vi "Config DMM.vi"(8 "error in (no error)":errorcluster, 10 "Load DMM Measurement":T1, 11 "IVI Refnum in":refnum<k15>) -> (0 "error out":errorcluster, 3 "IVI Refnum out":refnum<k15>)   [LabVIEW 2021, in "DMM T15.lvlib"]
uses:
  DMM T15.lvlib
  <instrlib>/niDMM/nidmm.llb/niDMM Function.ctl
  <instrlib>/niDMM/nidmm.llb/niDMM Configure Measurement Digits.vi
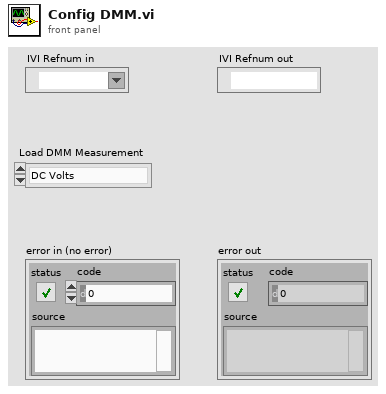
[diagram p1: front panel]
types:
  T1 = typedef "niDMM Function.ctl" = enum16{"DC Volts", "AC Volts", "DC Current", "AC Current", "2-wire Resistance", "4-wire Resistance", "Diode", "Frequency", "Period", "AC Volts DC Coupled", "Capacitance", "Inductance", "Temperature"}
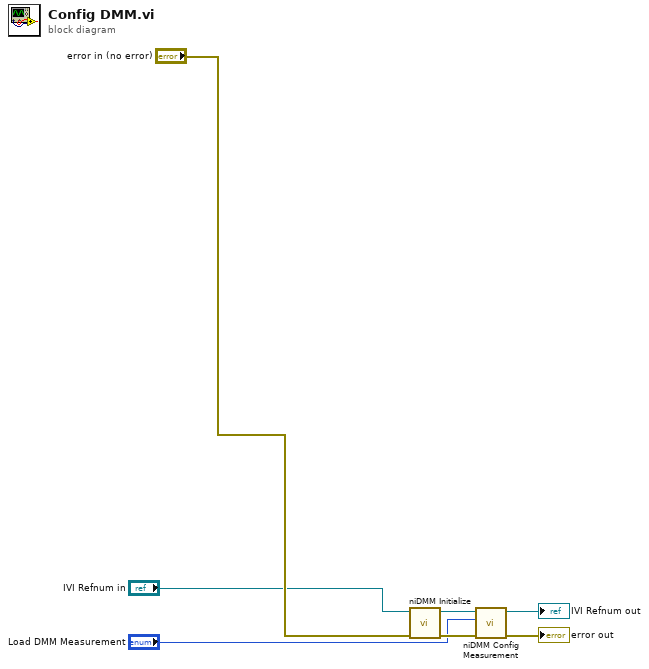
[diagram p0: block diagram]
diagram:
  n1 = call <instrlib>:"niDMM Initialize.vi"("error in (no error)"="error in (no error)", "Instrument Descriptor"="IVI Refnum in") -> ("error out"=w5:errorcluster, "instrument handle out"=w6:refnum<k15>)  [unwired: 8 in]
  n2 = call-poly <instrlib>:"niDMM Config Measurement.vi"("error in (no error)"=w5, "Function"="Load DMM Measurement", "instrument handle"=w6) -> ("error out"=→"error out":errorcluster, "instrument handle out"=→"IVI Refnum out":refnum<k15>)  [unwired: 7 in]
